vi "插入数组成员.vi"() -> ()   [LabVIEW 2010]
panel:
  out "插入后的数组":dbl[][](array[numeric]) format="%.2f"
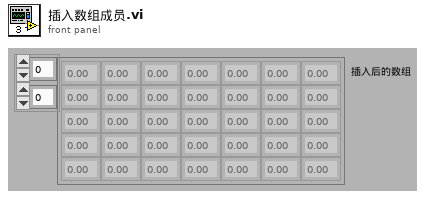
[diagram p1: front panel]
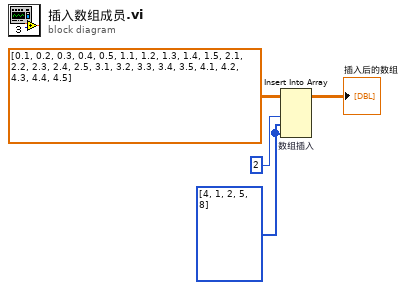
[diagram p0: block diagram]
diagram:
  w2 = i32[] [4, 1, 2, 5, 8]
  n1 = Insert Into Array "数组插入"(array=dbl[][] [[0.1, 0.2, 0.3, 0.4, 0.5], [1.1, 1.2, 1.3, 1.4, 1.5], [2.1, 2.2, 2.3, 2.4, 2.5], [3.1, 3.2, 3.3, 3.4, 3.5], [4.1, 4.2, 4.3, 4.4, 4.5]], index (col)=2 ("disabled index (col)"), new element #1=w2, new element #2=w2) -> (→"插入后的数组":dbl[][])  [unwired: 1 in]
